vi "PH_Beckhoff.get DA Values.vi"(0 "Digital Outputs":T1, 1 "Tags to get":string[](array[string])) -> (2 "Values":bool[](array[boolean]), 3 "Qualities":bool[](array[boolean]), 4 "Tags not found?":bool[](array[boolean]))   [LabVIEW 2014, in "PH_Beckhoff.lvlib"]
uses:
  PH_Beckhoff.lvlib
  PH_Beckhoff.Digital Outputs.ctl
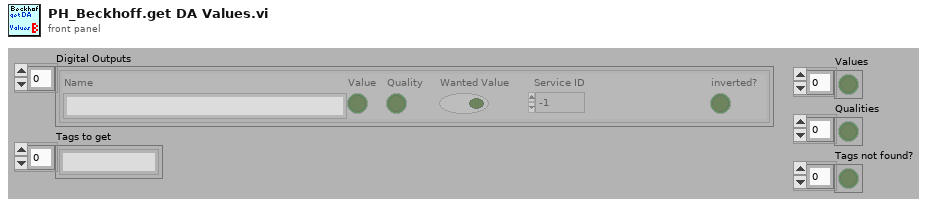
[diagram p1: front panel]
types:
  T1 = typedef "PH_Beckhoff.lvlib/PH_Beckhoff.Digital Outputs.ctl" = cluster{"Name":string, "Value":bool, "Quality":bool, "Wanted Value":bool, "Service ID":i32, "inverted?":bool}[]
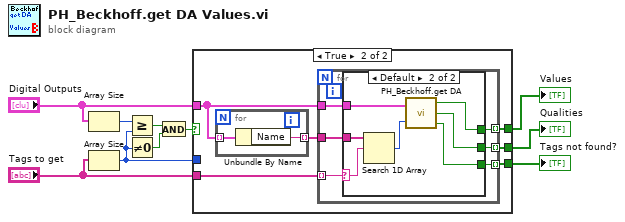
[diagram p0: block diagram]
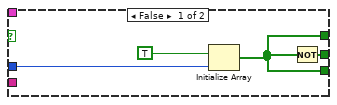
[diagram p2: hidden frame]
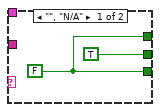
[diagram p3: hidden frame]
diagram:
  n1 = Array Size(array="Digital Outputs") -> (size(s)=w7:i32)
  n2 = Array Size(array="Tags to get") -> (size(s)=w4:i32)
  n3 = Greater Or Equal?(x=w7, y=w4) -> (x >= y?=w1:bool)
  n4 = Not Equal To 0?(x=w4) -> (x != 0?=w2:bool)
  n5 = And(x=w1, y=w2) -> (x .and. y?=w3:bool)
  n6 = case shown="True" w3 {
    tunnel: [w12 w20] -> w10
    tunnel: [w12 w19] -> w9
    tunnel: [w11 w17] -> w8
    tunnel: "Tags to get" -> [_ w15]
    tunnel: "Digital Outputs" -> [_ w16]
    tunnel: w4 -> [w13 _]
    frame False {
      n7 = Initialize Array(TRUE, w13) -> (w12:bool[])
      n8 = Not(x=w12) -> (.not. x?=w11:bool[])
    }
    frame True {
      n9 = for {
        tunnel: w16 -> [w22] mode=indexing
        tunnel: [w21] -> w18 mode=indexing
        n10 = Unbundle By Name(w22) -> ("Name"=w21:string)
      }
      n11 = for {
        tunnel: w16 -> [w28]
        tunnel: [w27] -> w17 mode=indexing
        tunnel: w18 -> [w26]
        tunnel: [w25] -> w20 mode=indexing
        tunnel: [w24] -> w19 mode=indexing
        tunnel: w15 -> [w23] mode=indexing
        n12 = case shown="Default" w23 {
          selector: w23 -> [_ w36]
          tunnel: w28 -> [_ w35]
          tunnel: [TRUE ("Quality") w32] -> w27
          tunnel: w26 -> [_ w37]
          tunnel: [w30 w31] -> w25
          tunnel: [w30 w33] -> w24
          frame "", "N/A" {
            w30 = FALSE
          }
          frame Default {
            n13 = Search 1D Array(1D array=w37, element=w36) -> (index of element=w34:i32)  [unwired: 1 in]
            n14 = call "PH_Beckhoff.get DA.vi"("Digital Outputs"=w35, "index of element"=w34) -> ("Value"=w33:bool, "Quality"=w32:bool, "Tag not found"=w31:bool)
          }
        }
      }
    }
  }
  "Tags not found?" <- w10
  "Values" <- w9
  "Qualities" <- w8
